vi "AimTIFKATS Controller.vi"(8 "error in":errorcluster) -> ()   [LabVIEW 2023]
doc: "This VI executes continuously carrying out the current operation and responding to updates or new operations. It will often contain the timing or control code that is difficult to place directly in TeleOp. This VI generally opens all sensors and motors and isolates the rest of the robot code from knowing how the operations are carried out."
uses:
  <vilib>/Rock Robotics/WPI/Framework/Completion Status.ctl
  AimTIFKATS Setpoints.ctl
  AimTIFKATS Operations.ctl
  <vilib>/Rock Robotics/WPI/ThirdParty/REV Robotics/REVLib/Typedef/Spark MAX Control Type.ctl
  <vilib>/Rock Robotics/Network Tables/NT Write Boolean.vi
panel:
  in  "TIFKATS offsets":dbl
  out "Applied Output":dbl=0.09323404644917142
  in  "PID Constants":T1={"P Gain"=9.0, "I Gain"=0.0, "D Gain"=0.0, "F Gain"=0.0, "I Zone"=0.0, "Min Output"=-1.0, "Max Output"=1.0}
  in  "Interactive Values":T2
  out "Current\nCmd":string="Started at  13:52:24.261\nDefault: Reserve,  S 0.0, D 0.000000"
  in  "Buttons":cluster{"Execute Cmd":bool, "Abort Cmd":bool}
  out "Command Timing":cluster{"Start Time (ms)":u32, "Iterations":i32}={"Start Time (ms)"=1167233, "Iterations"=0}
  out "Status":T4
  # "Tip: It may be helpful to observe inputs and sensor values.\nYou may also want to display tuning or debugging controls."
  # "Interactive Command: You may fill in the settings for a command\nand schedule it with the Execute button. You can observe and abort\nany command while fine tuning the code for the controller."
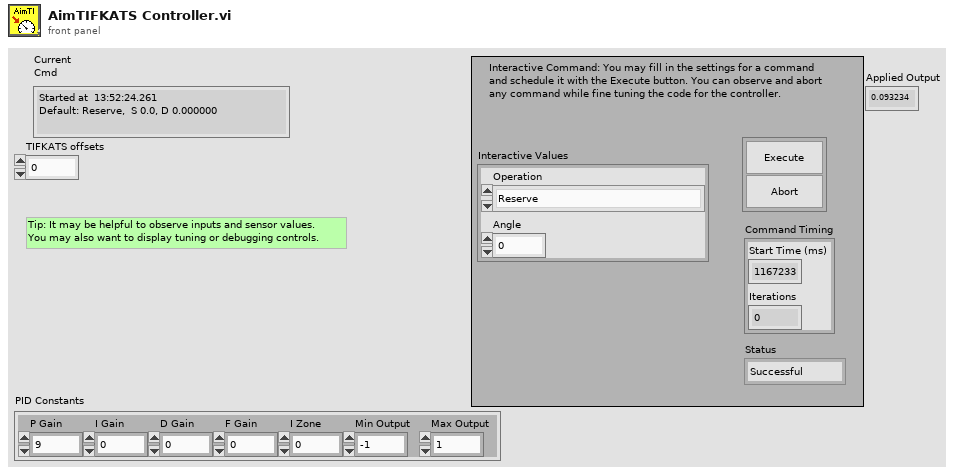
[diagram p1: front panel]
types:
  T1 = cluster{"P Gain":dbl, "I Gain":dbl, "D Gain":dbl, "F Gain":dbl, "I Zone":dbl, "Min Output":dbl, "Max Output":dbl}
  T2 = typedef "AimTIFKATS Setpoints.ctl" = cluster{"Operation":T3, "Angle":dbl}
  T3 = typedef "AimTIFKATS Operations.ctl" = enum16{"Reserve", "Read Current", "Immediate", "Angle up", "Angle down", "Angle to angle", "Stop rotate"}
  T4 = typedef "Completion Status.ctl" = enum16{"Successful", "Aborted", "Incomplete"}
  T5 = typedef "Command Status Info.ctl" = cluster{"Name":string, "Status":T4, "notifier out":T6}
  T6 = typedef "Completion Notifier.ctl" = refnum<notifier>
  T7 = cluster{"Current Command":T2, "Command Timing":cluster{"Start Time (ms)":u32, "Iterations":i32}, "Command Arguments":cluster{"Command Info":T5, "Description":string, "Default Command":T2, "queue out":refnum<queue>, "Subsystem Name":string}}
  T8 = typedef "Spark MAX Control Type.ctl" = enum16{"Percent VBus", "Voltage", "Velocity", "Position", "Smart Motion", "Current", "Smart Velocity"}
  T9 = typedef "WPI_MotorControlDeviceRef.ctl" = cluster{"DeviceStatus":errorcluster, "Type":T10, "PWM":cluster{"PWM Channel":T11, "DeadBand":T12}, "CAN":cluster{"Device Number":u8, "SetOutput VI Ref":variant, "GetOutput VI Ref":variant, "Enable VI Ref":variant, "Disable VI Ref":variant, "Data":variant}, "Invert":bool, "DIO PWM":cluster{"PWM \"Enable\" Channel":T11, "DIOChannel":T13, "PWM Rate":dbl}}
  T10 = typedef "WPI_MotorControlType.ctl" = enum16{"PWM", "CAN", "DIO PWM"}
  T11 = typedef "FPGA_DIOPWMChannel.ctl" = enum8{"PWM 0", "PWM 1", "PWM 2", "PWM 3", "PWM 4", "PWM 5", "PWM 6", "PWM 7", "PWM 8", "PWM 9", "PWM MXP 0", "PWM MXP 1", "PWM MXP 2", "PWM MXP 3", "PWM MXP 4", "PWM MXP 5", "PWM MXP 6", "PWM MXP 7", "PWM MXP 8", "PWM MXP 9", "Invalid"}
  T12 = typedef "WPI_PWMDeadband.ctl" = cluster{"Name":string, "maxPositivePwm":i32, "minPositivePwm":i32, "centerPwm":i32, "maxNegativePwm":i32, "minNegativePwm":i32, "angularRange":u16}
  T13 = typedef "FPGA_DIOChannel.ctl" = enum8{"DIO 0", "DIO 1", "DIO 2", "DIO 3", "DIO 4", "DIO 5", "DIO 6", "DIO 7", "DIO 8", "DIO 9", "DIO MXP 0", "DIO MXP 1", "DIO MXP 2", "DIO MXP 3", "DIO MXP 4", "DIO MXP 5", "DIO MXP 6", "DIO MXP 7", "DIO MXP 8", "DIO MXP 9", "DIO MXP 10", "DIO MXP 11", "DIO MXP 12", "DIO MXP 13", "DIO MXP 14", "DIO MXP 15", "SPI Port CS1", "SPI Port CS2", "SPI Port CS3", "SPI Port MISO", "SPI Port MOSI", "Invalid"}
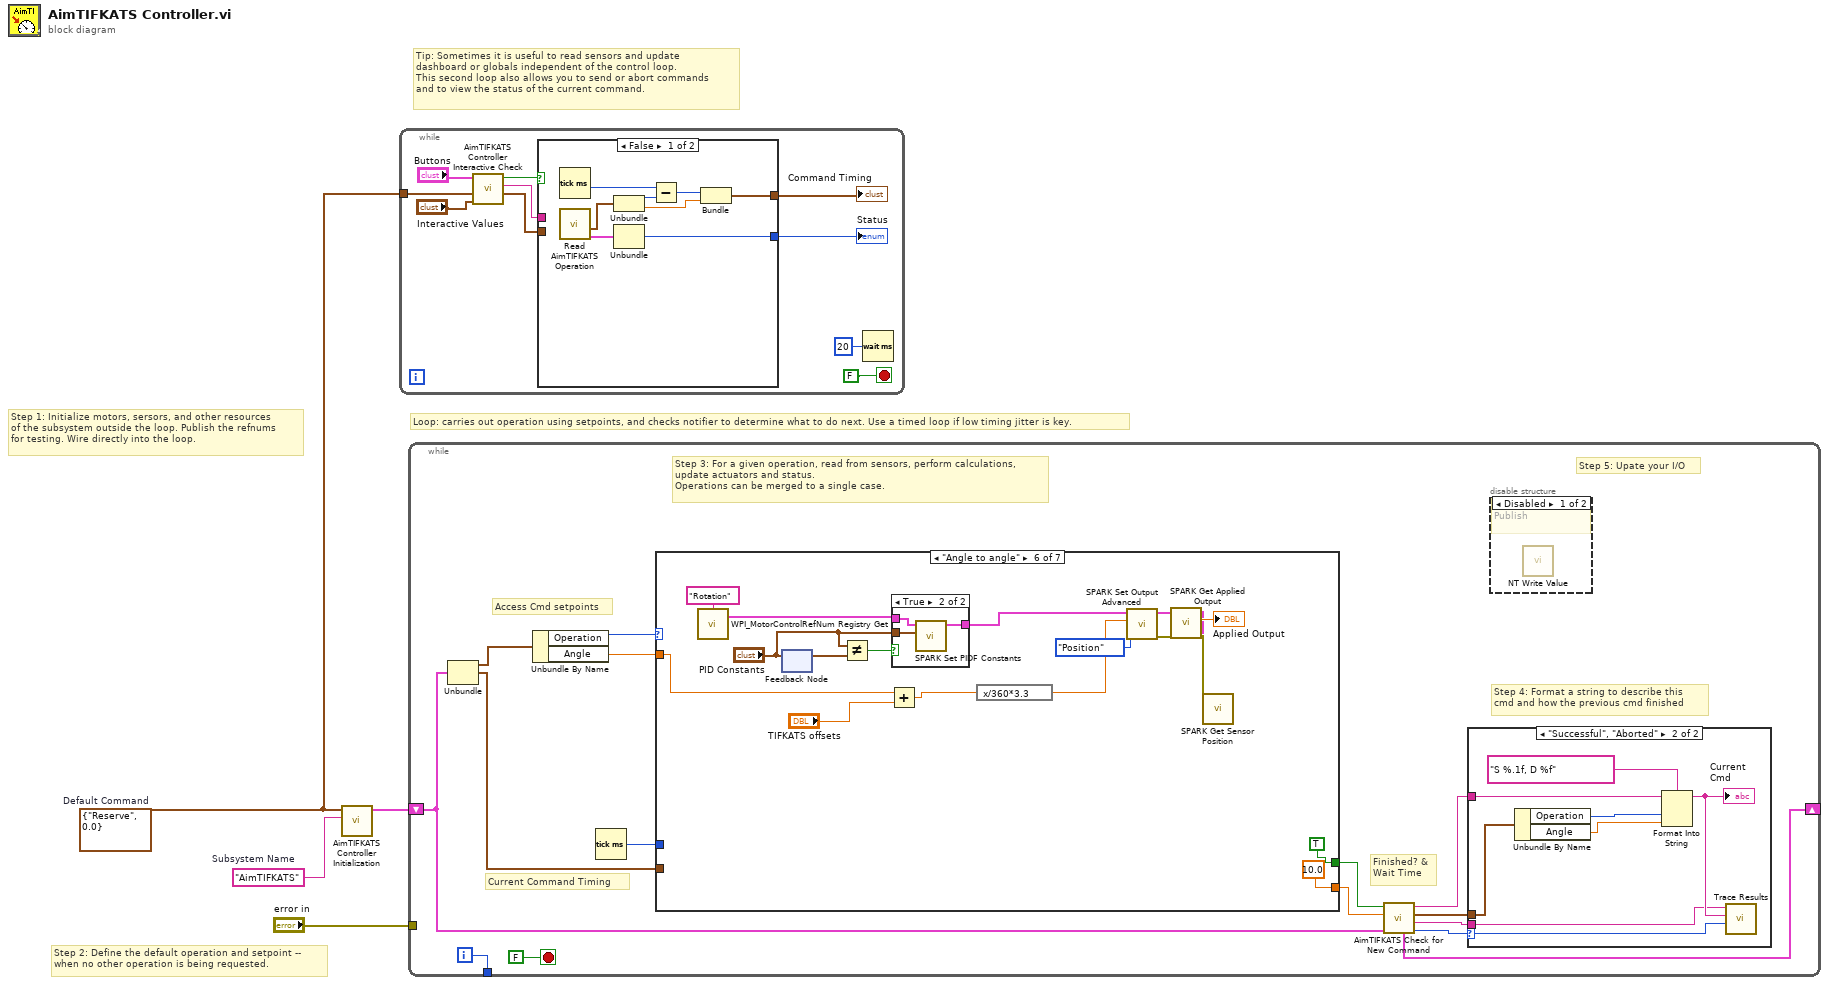
[diagram p0: block diagram]
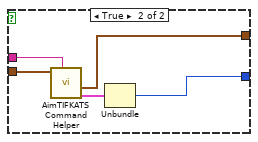
[diagram p2: hidden frame]
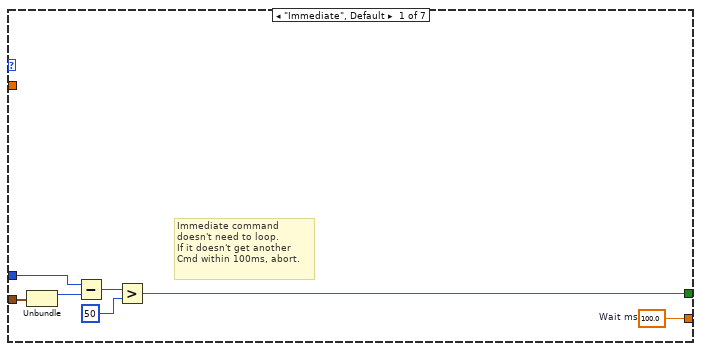
[diagram p5: hidden frame]
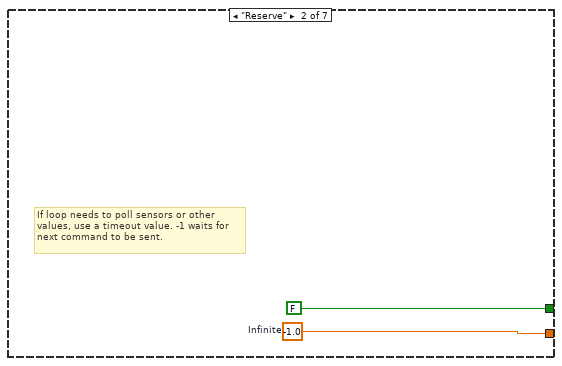
[diagram p6: hidden frame]
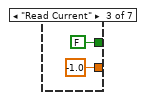
[diagram p7: hidden frame]
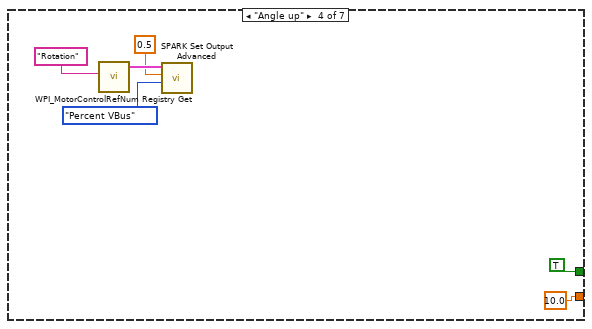
[diagram p8: hidden frame]
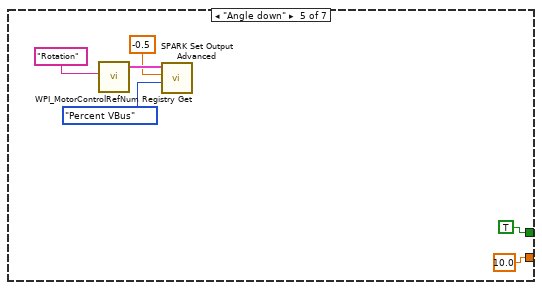
[diagram p9: hidden frame]
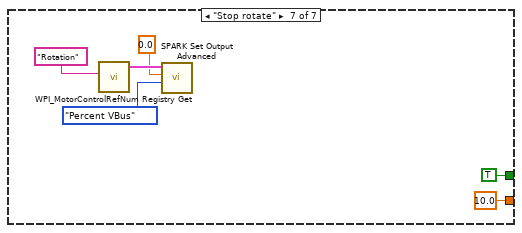
[diagram p11: hidden frame]
diagram:
  w1 = T2 {"Operation"=enum."Reserve", "Angle"=0.0}  # Default Command
  w2 = "AimTIFKATS"  # Subsystem Name
  # "Tip: Sometimes it is useful to read sensors and update\ndashboard or globals independent of the control loop.\nThis second loop also allows you to send or abort commands\nand to view the status of the current command."
  # "Step 2: Define the default operation and setpoint --\nwhen no other operation is being requested."
  # "Step 1: Initialize motors, sersors, and other resources\nof the subsystem outside the loop. Publish the refnums\nfor testing. Wire directly into the loop."
  # "Loop: carries out operation using setpoints, and checks notifier to determine what to do next. Use a timed loop if low timing jitter is key."
  n1 = call "AimTIFKATS Controller Initialization.vi"("Subsystem Name"=w2, "Default Command"=w1) -> ("Current Command"=w3:T7)  [unwired: 9 in]
  n2 = while {
    tunnel: w1 -> [w11]
    stop <- FALSE stop-if-true
    n3 = call "AimTIFKATS Controller Interactive Check.vi"("Interactive Command in"="Interactive Values", "Default Command"=w11, "Buttons"="Buttons") -> ("Interactive Command out"=w8:T2, "Trace String"=w9:string, "Schedule"=w10:bool)  [unwired: 6 in]
    n4 = case shown="False" w10 {
      tunnel: [w22 w27] -> w7
      tunnel: w8 -> [_ w25]
      tunnel: [w18 w23] -> w6
      tunnel: w9 -> [_ w26]
      frame False {
        n5 = Tick Count (ms)() -> (millisecond timer value=w17:u32)
        n6 = call "Read AimTIFKATS Operation.vi"() -> ("Command Info"=w15:T5, "SubSystem Data"=w16:T2)  [unwired: 9 in, 1 out]
        n7 = Unbundle(w16) -> ("Operation"=w21:T3, "Angle"=w19:dbl)
        n8 = Unbundle(w15) -> ("Status"=w22:T4)  [unwired: 2 out]
        n9 = Subtract(x=w17, y=w21) -> (x-y=w20:u32)
        n10 = Bundle(w20, "Angle"=w19) -> (w18:cluster{u32, "Angle":dbl})  [unwired: 1 in]
      }
      frame True {
        n11 = call "AimTIFKATS Command Helper.vi"("Description"=w26, "SubSystem Data"=w25) -> ("Command Info Out"=w24:T5, "Command Timing"=w23:cluster{"Start Time (ms)":u32, "Iterations":i32})  [unwired: 7 in, 1 out]
        n12 = Unbundle(w24) -> ("Status"=w27:T4)  [unwired: 2 out]
      }
    }
    "Status" <- w7
    "Command Timing" <- w6
    n13 = Wait (ms)(milliseconds to wait=u32 20) -> ()  [unwired: 1 out]
  }
  n14 = while {
    shift-right: [w35] -> _
    shift-left: w3 -> [w28]
    tunnel: [w41] -> _
    tunnel: "error in" -> [_]
    i -> [w41]
    stop <- FALSE stop-if-true
    # "Step 5: Upate your I/O"
    # "Step 4: Format a string to describe this\ncmd and how the previous cmd finished"
    # "Current Command Timing"
    # "Access Cmd setpoints"
    # "Finished? &\nWait Time"
    # "Step 3: For a given operation, read from sensors, perform calculations,\nupdate actuators and status.\nOperations can be merged to a single case."
    n15 = Unbundle(w28) -> ("Current Command"=w40:T2, "Command Timing"=w36:cluster{"Start Time (ms)":u32, "Iterations":i32})  [unwired: 1 out]
    n16 = Unbundle By Name(w40) -> ("Operation"=w39:T3, "Angle"=w38:dbl)
    n17 = Tick Count (ms)() -> (millisecond timer value=w37:u32)
    n18 = case shown="\"Angle to angle\"" w39 {
      tunnel: [w57 w59 -1.0 ("Infinite") 10.0 ("Infinite") 10.0 ("Infinite") 10.0 ("Infinite") 10.0 ("Infinite")] -> w33
      tunnel: [w51 FALSE ("ignore previous (F)") FALSE ("ignore previous (F)") TRUE ("ignore previous (F)") TRUE ("ignore previous (F)") TRUE ("ignore previous (F)") TRUE ("ignore previous (F)")] -> w34
      tunnel: w36 -> [w53 _ _ _ _ _ _]
      tunnel: w38 -> [_ _ _ _ _ w76 _]
      tunnel: w37 -> [w52 _ _ _ _ _ _]
      frame "Immediate", Default {
        w57 = 100.0  # Wait ms
        # "Immediate command\ndoesn't need to loop.\nIf it doesn't get another\nCmd within 100ms, abort."
        n19 = Unbundle(w53) -> ("Start Time (ms)"=w56:u32)  [unwired: 1 out]
        n20 = Subtract(x=w52, y=w56) -> (x-y=w55:u32)
        n21 = Greater?(x=w55, y=u8 50 ("Left Motor")) -> (0:w51:bool)
      }
      frame "Reserve" {
        w59 = -1.0  # Infinite
        # "If loop needs to poll sensors or other\nvalues, use a timeout value. -1 waits for\nnext command to be sent."
      }
      frame "Read Current" {
      }
      frame "Angle up" {
        n22 = call <vilib>:"WPI_MotorControlRefNum Registry Get.vi"("refnum name"="Rotation") -> ("MotorControlDevRef"=w66:T9)  [unwired: 9 in, 1 out]
        n23 = call <vilib>:"SPARK Set Output Advanced.vi"("Control Mode"=Spark_MAX_Control_Type."Percent VBus", "Setpoint"=0.5 ("Output"), "MotorControlDevRef"=w66) -> ()  [unwired: 7 in, 2 out]
      }
      frame "Angle down" {
        n24 = call <vilib>:"WPI_MotorControlRefNum Registry Get.vi"("refnum name"="Rotation") -> ("MotorControlDevRef"=w72:T9)  [unwired: 9 in, 1 out]
        n25 = call <vilib>:"SPARK Set Output Advanced.vi"("Control Mode"=Spark_MAX_Control_Type."Percent VBus", "Setpoint"=-0.5 ("Output"), "MotorControlDevRef"=w72) -> ()  [unwired: 7 in, 2 out]
      }
      frame "Angle to angle" {
        n26 = call <vilib>:"WPI_MotorControlRefNum Registry Get.vi"("refnum name"="Rotation") -> ("MotorControlDevRef"=w89:T9)  [unwired: 9 in, 1 out]
        n27 = feedback #1() -> (w86:T1)  [unwired: 1 in]
        n28 = feedback-in #1("PID Constants") -> ()
        n29 = Not Equal?(x="PID Constants", y=w86) -> (x != y?=w85:bool)
        n30 = Add(x=w76, y="TIFKATS offsets") -> (x+y=w75:dbl)
        n31 = case shown="True" w85 {
          tunnel: "PID Constants" -> [_ w95]
          tunnel: w89 -> [w92 w94]
          tunnel: [w92 w93] -> w88
          frame False {
          }
          frame True {
            n32 = call <vilib>:"SPARK Set PIDF Constants.vi"("PID Constants"=w95, "MotorControlDeviceRef"=w94) -> ("MotorControlDeviceRef"=w93:T9)  [unwired: 8 in, 1 out]
          }
        }
        n33 = expression code="x/360*3.3"(w75) -> (w84:dbl)
        n34 = call <vilib>:"SPARK Set Output Advanced.vi"("Control Mode"=Spark_MAX_Control_Type."Position", "Setpoint"=w84, "MotorControlDevRef"=w88) -> ("error out"=w83:errorcluster, "MotorControlDevRef"=w82:T9)  [unwired: 7 in]
        n35 = call <vilib>:"SPARK Get Applied Output.vi"("error in (no error)"=w83, "MotorControlDevRef in"=w82) -> ("error out"=w80:errorcluster, "Applied Output"=→"Applied Output":dbl, "MotorControlDevRef out"=w79:T9)  [unwired: 6 in, 1 out]
        n36 = call <vilib>:"SPARK Get Sensor Position.vi"("error in (no error)"=w80, "MotorControlDevRef in"=w79) -> ()  [unwired: 6 in, 4 out]
      }
      frame "Stop rotate" {
        n37 = call <vilib>:"WPI_MotorControlRefNum Registry Get.vi"("refnum name"="Rotation") -> ("MotorControlDevRef"=w100:T9)  [unwired: 9 in, 1 out]
        n38 = call <vilib>:"SPARK Set Output Advanced.vi"("Control Mode"=Spark_MAX_Control_Type."Percent VBus", "Setpoint"=0.0 ("Output"), "MotorControlDevRef"=w100) -> ()  [unwired: 7 in, 2 out]
      }
    }
    n39 = call "AimTIFKATS Check for New Command.vi"("Current Command"=w28, "Wait time (ms)"=w33, "Finished?"=w34) -> ("Completion"=w29:T4, "Subsystem Name"=w30:string, "Current Command"=w31:T2, "Initial Trace String"=w32:string, "NextCommand"=w35:T7)  [unwired: 4 in]
    n40 = case shown="\"Successful\", \"Aborted\"" w29 {
      selector: w29 -> [_ w50]
      tunnel: w32 -> [_ w46]
      tunnel: w31 -> [_ w47]
      tunnel: w30 -> [_ w44]
      frame "Incomplete", Default {
        # "Continuing current command"
      }
      frame "Successful", "Aborted" {
        # "Report and setup for next command"
        n41 = Unbundle By Name(w47) -> ("Operation"=w49:T3, "Angle"=w43:dbl)
        n42 = Format Into String(format string="S %.1f, D %f", initial string=w46, w49, w43) -> (resulting string=w45:string)  [unwired: 1 in, 1 out]
        "Current\nCmd" <- w45
        n43 = call <vilib>:"Trace Results.vi"("Status of previous command"=w50, "Description"=w45, "Subsystem"=w44) -> ()  [unwired: 9 in]
      }
    }
    n44 = disable-structure shown="Disabled" {
      frame Disabled {
        # "Publish"
        n45 = call-poly <vilib>:"NT Write Value.vi"() -> ()  [unwired: 11 in, 1 out]
      }
      frame Enabled {
      }
    }
  }
